vi "Wait_Test.vi"(8 "error in (no error)":errorcluster caption="entrée d'erreur (pas d'erreur)", 11 "Test (Default) en entrée":refnum<class "Sequencer (Default).lvclass">) -> (0 "error out":errorcluster caption="sortie d'erreur", 3 "Test (Default) en sortie":refnum<class "Sequencer (Default).lvclass">)   [LabVIEW 2020, in "Library Core.lvlib" / "Sequencer (Default).lvclass"]
uses:
  Sequencer (Default).lvclass
  Sequencer (Default).lvclass/Sequencer (Default).ctl
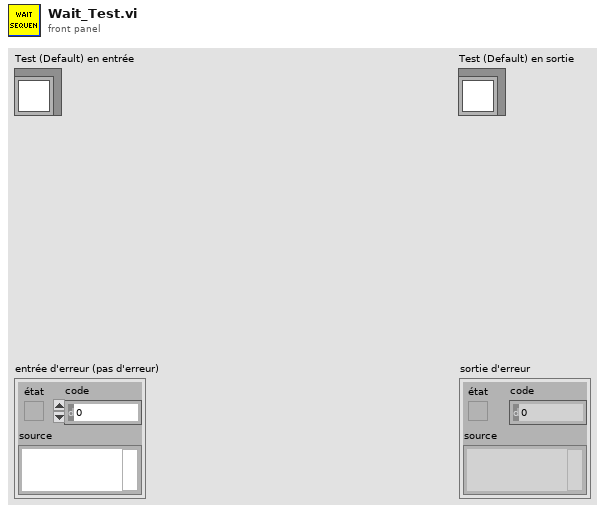
[diagram p1: front panel]
types:
  T1 = typedef "Library Commun.lvlib/Commande Value Type.ctl" = enum16{"None", "String", "Number", "Timestamp", "Boolean", "Array"}
  T2 = typedef "Library Commun.lvlib/Commande Type Test.ctl" = enum16{"Function", "Test", "Calculation"}
  T3 = cluster{"Main Test":string, "Name Test":string, "StartOfTest":string, "Value":string, "Limit_Low":string, "Limit_High":string, "Result":bool, "Fatal_Test":bool, "NbRetry":dbl, "EndOfTest":string, "Error":string, "TypeValue":T1, "Type Test":T2}[][]
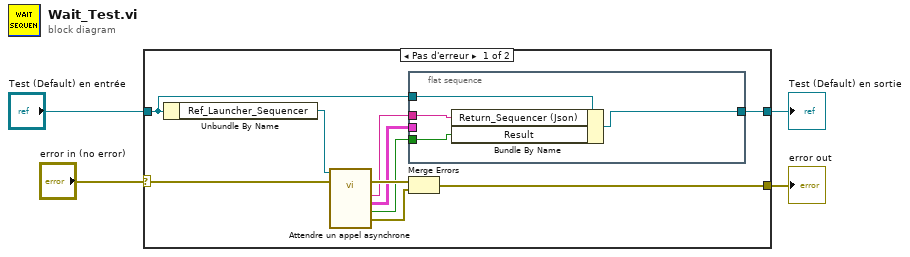
[diagram p0: block diagram]
diagram:
  n1 = case shown="Pas d'erreur" "error in (no error)" {
    selector: "error in (no error)" -> [w13 w20]
    tunnel: [w5 w20] -> w2
    tunnel: [w10 w19] -> w1
    tunnel: "Test (Default) en entrée" -> [w8 w19]
    frame No Error {
      n2 = Unbundle By Name(w8) -> ("Ref_Launcher_Sequencer"=w14:refnum<vi>)
      n3 = call-by-ref "Attendre un appel asynchrone"(reference=w14, error in=w13) -> (error out=w12:errorcluster, 0:"error out"=w11:errorcluster, "Result"=w6:bool, "Result Sequence"=w7:T3, "Json_String"=w9:string)  [unwired: 8 in, 1 out]
      n4 = flat-sequence {
        tunnel: [w16] -> w10
        tunnel: w9 -> [w18]
        tunnel: w8 -> [w17]
        tunnel: w7 -> [_]
        tunnel: w6 -> [w15]
        frame #0 {
          n5 = Bundle By Name(cluster=w17, "Return_Sequencer (Json)"=w18, "Result"=w15) -> (w16:refnum<class "Sequencer (Default).lvclass">)
        }
      }
      n6 = Merge Errors(w12, w11) -> (w5:errorcluster)
    }
    frame Error {
    }
  }
  "error out" <- w2
  "Test (Default) en sortie" <- w1
